vi "Check For Response.vi"(8 "error in (no error)":errorcluster, 10 "id String":string, 11 "Server in":refnum<class "JSONRPC Server.lvclass">) -> (0 "error out":errorcluster, 1 "found":bool, 2 "response string":string, 3 "Server out":refnum<class "JSONRPC Server.lvclass">)   [LabVIEW 2016, in "JSONRPC Server.lvclass"]
doc: "Check if a Response with the id String is on the RPC Server. For numeric ids, use the string representation of the number. For String ids, place the id string in quotes. For Example:\n\n(DBL) 1 = 1\n(STR) 1 = \"1\""
uses:
  JSONRPC Server.lvclass
  Get Response Tree.vi
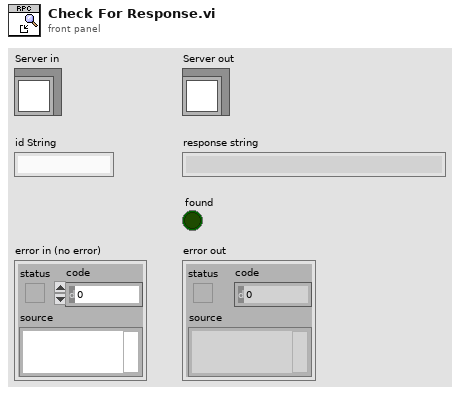
[diagram p1: front panel]
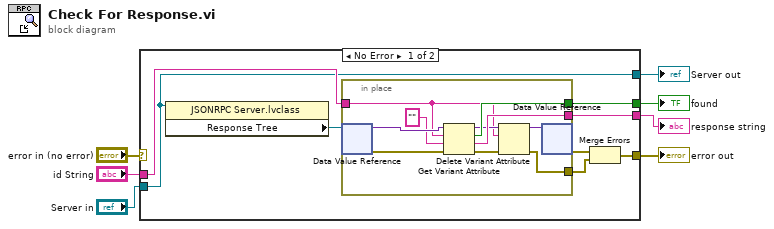
[diagram p0: block diagram]
diagram:
  n1 = case shown="No Error" "error in (no error)" {
    selector: "error in (no error)" -> [_ w27]
    tunnel: [w11 w27] -> w6
    tunnel: [w9 w26] -> w4
    tunnel: "Server in" -> [w9 w26]
    tunnel: "id String" -> [w15 _]
    tunnel: [w14 _] -> w2
    tunnel: [w10 _] -> w1
    frame No Error {
      n2 = property class="JSONRPC Server.lvclass"(reference=w9) -> ("Response Tree"=w8:refnum<data-value>)  [unwired: 1 in, 2 out]
      n3 = in-place {
        in-place-border: w15 -> [w18]
        in-place-border: [w24] -> w14
        in-place-border: [w16] -> w12
        in-place-border: [w22] -> w10
        n4 = in-place-dvr #1(w8) -> (w25:variant, w23:errorcluster)
        n5 = Get Variant Attribute(Variant=w25, name=w18, default value (empty Variant)="", error in=w23) -> (duplicate Variant=w20:variant, found=w24:bool, value=w22:string, error out=w17:errorcluster)
        n6 = Delete Variant Attribute(4:w17, 6:w18, 7:w20) -> (0:w16:errorcluster, 3:w19:variant)  [unwired: 1 out]
        n7 = in-place-dvr #1(w19) -> (w13:errorcluster)  [unwired: 1 out]
      }
      n8 = Merge Errors(w13, w12) -> (w11:errorcluster)
    }
    frame Error {
    }
  }
  "error out" <- w6
  "Server out" <- w4
  "found" <- w2
  "response string" <- w1
